vi "CH_LM Config Resolution.vi"(0 "Meter Index":i32, 2 "Probe Type":T2=enum."Thermopile", 3 "Resolution (3 1/2)":T1, 5 "error in (no error)":errorcluster, 7 "Timeout / ms (3000)":i32=3000, 8 "Action (query)":bool, 9 "Lock Timeout / ms (1000)":i32=1000) -> (11 "Lock timed out":bool, 14 "Meter Index":i32, 17 "Resolution (3 1/2)":T1, 19 "error out":errorcluster)   [LabVIEW 2012, in "CH_LM.lvlib"]
doc: "Front panel numeric display resolution will is configurable from among the following set of display digit counts: 3½, 4½, 5½, and 6½."
uses:
  CH_LM.lvlib
  CH_LM ProbeType.ctl
  CH_LM Numeric Resolution.ctl
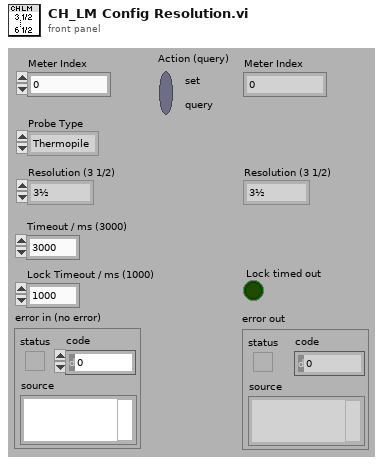
[diagram p1: front panel]
types:
  T1 = typedef "CH_LM.lvlib/CH_LM Numeric Resolution.ctl" = enum16{"3½", "4½", "5½", "6½"}
  T2 = typedef "CH_LM.lvlib/CH_LM ProbeType.ctl" = enum16{"None", "Thermopile", "Pyroelectric", "Optical"}
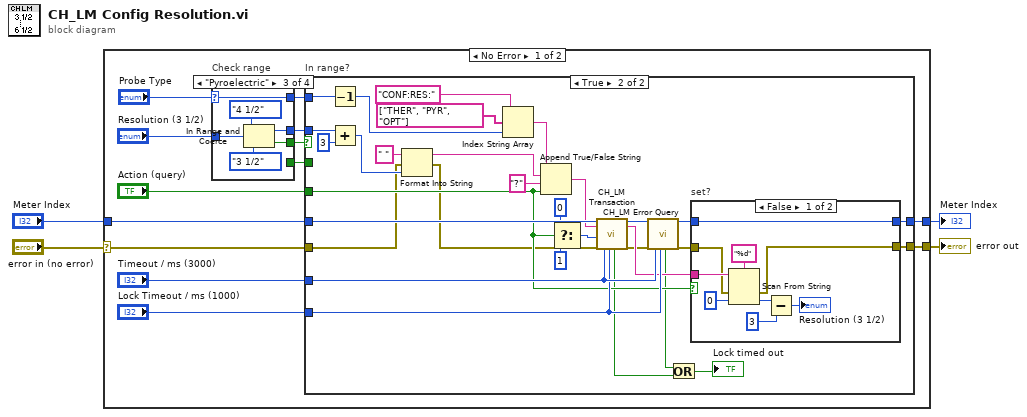
[diagram p0: block diagram]
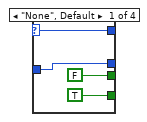
[diagram p2: hidden frame]
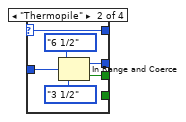
[diagram p3: hidden frame]
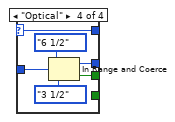
[diagram p4: hidden frame]
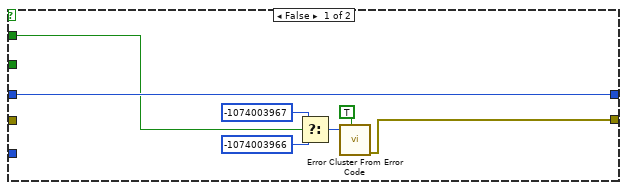
[diagram p5: hidden frame]
diagram:
  n1 = case shown="No Error" "error in (no error)" {
    selector: "error in (no error)" -> [w17 w90]
    tunnel: [w15 w90] -> w4
    tunnel: "Meter Index" -> [w16 w89]
    tunnel: [w14 w89] -> w1
    frame No Error {
      n2 = case "Check range" shown="\"Pyroelectric\"" "Probe Type" {
        selector: "Probe Type" -> [w18 w22 w28 w34]
        tunnel: [w19 w27 w33 w39] -> w11
        tunnel: [FALSE w26 w32 w38] -> w9
        tunnel: "Resolution (3 1/2)" -> [w19 w25 w31 w37]
        tunnel: [TRUE _ _ _] -> w6
        tunnel: [w18 w22 w28 w34] -> w5
        frame "None", Default {
        }
        frame "Thermopile" {
          n3 = In Range and Coerce(upper limit=enum16{"3 1/2", "4 1/2", "5 1/2", "6 1/2"}."6 1/2", x=w25, lower limit=enum16{"3 1/2", "4 1/2", "5 1/2", "6 1/2"}."3 1/2") -> (coerced(x)=w27:u16, In Range?=w26:bool)
        }
        frame "Pyroelectric" {
          n4 = In Range and Coerce(upper limit=enum16{"3 1/2", "4 1/2", "5 1/2", "6 1/2"}."4 1/2", x=w31, lower limit=enum16{"3 1/2", "4 1/2", "5 1/2", "6 1/2"}."3 1/2") -> (coerced(x)=w33:u16, In Range?=w32:bool)
        }
        frame "Optical" {
          n5 = In Range and Coerce(upper limit=enum16{"3 1/2", "4 1/2", "5 1/2", "6 1/2"}."6 1/2", x=w37, lower limit=enum16{"3 1/2", "4 1/2", "5 1/2", "6 1/2"}."3 1/2") -> (coerced(x)=w39:u16, In Range?=w38:bool)
        }
      }
      n6 = case "In range?" shown="True" w9 {
        tunnel: w17 -> [_ w48]
        tunnel: w16 -> [w46 w77]
        tunnel: [w44 w76] -> w15
        tunnel: [w46 w75] -> w14
        tunnel: "Timeout / ms (3000)" -> [_ w74]
        tunnel: "Lock Timeout / ms (1000)" -> [_ w73]
        tunnel: "Action (query)" -> [_ w72]
        tunnel: w11 -> [_ w58]
        tunnel: w6 -> [w43 _]
        tunnel: w5 -> [_ w56]
        frame False {
          n7 = Select(t=-1074003967 ("error code (0)"), s=w43, f=-1074003966 ("error code (0)")) -> (s? t:f=w41:i32)
          n8 = call <vilib>:"Error Cluster From Error Code.vi"("show call chain? (False)"=TRUE, "error code (0)"=w41) -> ("error out"=w44:errorcluster)  [unwired: 1 in, 6 out]
        }
        frame True {
          n9 = Decrement(x=w56) -> (x-1=w53:T2)
          n10 = Add(x=w58, y=3) -> (x+y=w50:i32)
          n11 = Format Into String(initial string=" ", error in=w48, w50) -> (resulting string=w49:string, error out=w47:errorcluster)  [unwired: 1 in]
          n12 = Index String Array(1:w53, 2:string[] ["THER", "PYR", "OPT"], 3:"CONF:RES:" ("Command String")) -> (0:w52:string)
          n13 = Append True/False String(1:w72, 2:"?" ("true string"), 3:w49, 4:w52) -> (0:w59:string)
          n14 = Select(t=0, s=w72, f=1 ("NofStrings (-1:all)")) -> (s? t:f=w68:i32)
          n15 = call "CH_LM Transaction.vi"("Meter Index"=w77, "Command String"=w59, "NofStrings (-1:all)"=w68, "error in (no error)"=w47, "Timeout / ms (3000)"=w74, "Lock Timeout / ms (1000)"=w73) -> ("Lock timed out"=w61:bool, "Meter Index"=w66:i32, "Response"=w71:string, "error out"=w64:errorcluster)  [unwired: 10 out]
          n16 = call "CH_LM Error Query.vi"("Meter Index"=w66, "error in (no error)"=w64, "Timeout / ms (3000)"=w74, "Lock Timeout / ms (1000)"=w73) -> ("Lock timed out"=w62:bool, "Meter Index"=w65:i32, "error out"=w63:errorcluster)  [unwired: 13 out]
          n17 = Or(x=w62, y=w61) -> (x .or. y?=→"Lock timed out":bool)
          n18 = case "set?" shown="False" w72 {
            tunnel: w71 -> [w86 _]
            tunnel: w63 -> [w85 w88]
            tunnel: [w84 w88] -> w76
            tunnel: w65 -> [w81 w87]
            tunnel: [w81 w87] -> w75
            frame False {
              n19 = Scan From String(format string="%d", input string=w86, error in=w85, default 1=u16 0 ("default value 1")) -> (error out=w84:errorcluster, output 1=w80:u16)  [unwired: 1 in, 2 out]
              n20 = Subtract(x=w80, y=u16 3) -> (x-y=→"Resolution (3 1/2)":u16)
            }
            frame True {
            }
          }
        }
      }
    }
    frame Error {
    }
  }
  "error out" <- w4
  "Meter Index" <- w1
